vi "Dispense.vi"() -> ()   [LabVIEW 2014]
uses:
  Dispenser Functions.ctl
panel:
  out "error out":errorcluster
  in  "error in (no error)":errorcluster
  in  "Bottom Pin":tag="B/PWM0"
  in  "Top Pin":tag="B/PWM0"
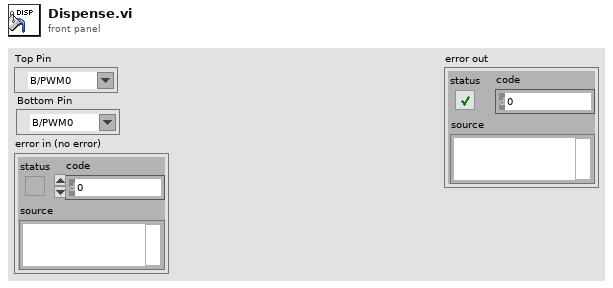
[diagram p1: front panel]
types:
  T1 = typedef "Dispenser Functions.ctl" = enum16{"Open Top", "Close Top", "Close Bottom", "Open Bottom"}
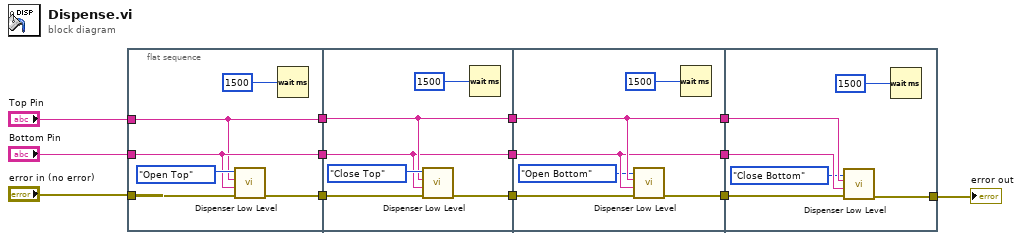
[diagram p0: block diagram]
diagram:
  n1 = flat-sequence {
    tunnel: "Bottom Pin" -> [w15]
    tunnel: [w15] -> w12
    tunnel: "Top Pin" -> [w14]
    tunnel: [w14] -> w8
    tunnel: "error in (no error)" -> [w18]
    tunnel: [w17] -> w5
    tunnel: w12 -> [w21]
    tunnel: [w21] -> w11
    tunnel: w8 -> [w22]
    tunnel: [w22] -> w7
    tunnel: w5 -> [w23]
    tunnel: [w20] -> w3
    tunnel: w11 -> [w29]
    tunnel: [w29] -> w10
    tunnel: w7 -> [w30]
    tunnel: [w30] -> w6
    tunnel: w3 -> [w27]
    tunnel: [w26] -> w2
    tunnel: w10 -> [w33]
    tunnel: w6 -> [w34]
    tunnel: w2 -> [w36]
    tunnel: [w35] -> w1
    frame #0 {
      n2 = call "Dispenser Low Level.vi"("error in (no error)"=w18, "Bottom Pin"=w15, "Top Pin"=w14, "Function"=Dispenser_Functions."Open Top") -> ("error out"=w17:errorcluster)  [unwired: 7 in]
      n3 = Wait (ms)(milliseconds to wait=u32 1500) -> ()  [unwired: 1 out]
    }
    frame #1 {
      n4 = call "Dispenser Low Level.vi"("error in (no error)"=w23, "Bottom Pin"=w21, "Top Pin"=w22, "Function"=Dispenser_Functions."Close Top") -> ("error out"=w20:errorcluster)  [unwired: 7 in]
      n5 = Wait (ms)(milliseconds to wait=u32 1500) -> ()  [unwired: 1 out]
    }
    frame #2 {
      n6 = call "Dispenser Low Level.vi"("error in (no error)"=w27, "Bottom Pin"=w29, "Top Pin"=w30, "Function"=Dispenser_Functions."Open Bottom") -> ("error out"=w26:errorcluster)  [unwired: 7 in]
      n7 = Wait (ms)(milliseconds to wait=u32 1500) -> ()  [unwired: 1 out]
    }
    frame #3 {
      n8 = call "Dispenser Low Level.vi"("error in (no error)"=w36, "Bottom Pin"=w33, "Top Pin"=w34, "Function"=Dispenser_Functions."Close Bottom") -> ("error out"=w35:errorcluster)  [unwired: 7 in]
      n9 = Wait (ms)(milliseconds to wait=u32 1500) -> ()  [unwired: 1 out]
    }
  }
  "error out" <- w1
